vi "Instrument Type ID.vi"() -> (1 "instrument type id":string="niDCPower")   [LabVIEW 2020, in "niDCPower Sessions.lvlib"]
uses:
  niDCPower Sessions.lvlib
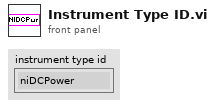
[diagram p1: front panel]
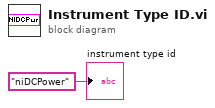
[diagram p0: block diagram]
diagram:
  "instrument type id" <- "niDCPower"
